vi "AutofocusToWire.vi"(4 "error in (no error)":errorcluster, 5 "Z position Guess":dbl, 6 "Session In":T1, 7 "controller in":refnum<k24>) -> (0 "error out":errorcluster, 1 "Z Position Feedback":dbl, 2 "Session Out":T1, 3 "controller out":refnum<k24>)   [LabVIEW 2016]
uses:
  C:/Users/sciollalab/Documents/Brandeis-BNL/LabVIEW_Codes/BNLStaveAssembly-Blueprint/Bin/Aerotech.A3200.dll
  BNLStaveAssembly-Blueprint/Bin/Aerotech.A3200.dll
  <vilib>/userdefined/High Color/IMAQdx.ctl
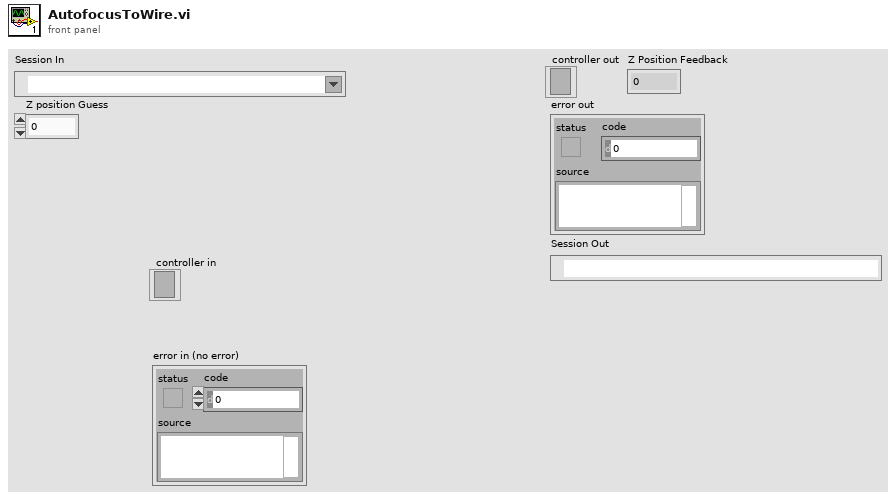
[diagram p1: front panel]
types:
  T1 = typedef "IMAQdx.ctl" = refnum<k21>
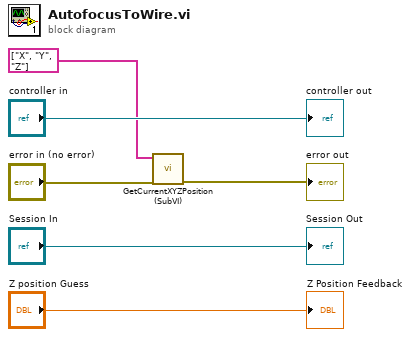
[diagram p0: block diagram]
diagram:
  n1 = call "GetCurrentXYZPosition (SubVI).vi"("error in (no error)"="error in (no error)", "Axes Names"=string[] ["X", "Y", "Z"]) -> ("error out"=→"error out":errorcluster)  [unwired: 4 in, 5 out]
  "controller out" <- "controller in"
  "Session Out" <- "Session In"
  "Z Position Feedback" <- "Z position Guess"
